vi "USB2XXX_LIN_Test.vi"() -> ()   [LabVIEW 2010]
panel:
  out "write return":i32
  out "pLINMsg out":T1
  out "read return":i32
  in  "pLINWiteMsg":T1={"ID"=2, "DataLen"=8, "Data[0]"=1, "Data[1]"=0, "Data[2]"=0, "Data[3]"=0, "Data[4]"=0, "Data[5]"=0, "Data[6]"=0, "Data[7]"=0, "Data[8]"=8}
  in  "pConfig":T2={"BaudRate"=19200, "CheckMode"=1, "MasterMode"=1, "BreakBits"=13}
  in  "Channel Index":u8(ring) items=["CH0"]
  in  "Device Index":i32(ring) items=["0", "1", "2", "3", "4", "5"]
  out "Flag(T:Write;F:Read)":bool=TRUE
  in  "stop":bool
  in  "Read":bool
  in  "Write":bool
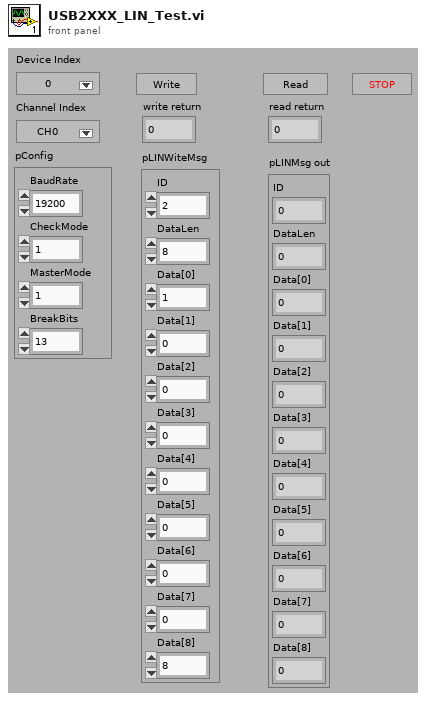
[diagram p1: front panel]
types:
  T1 = cluster{"ID":u8, "DataLen":u8, "Data[0]":u8, "Data[1]":u8, "Data[2]":u8, "Data[3]":u8, "Data[4]":u8, "Data[5]":u8, "Data[6]":u8, "Data[7]":u8, "Data[8]":u8}
  T2 = cluster{"BaudRate":u32, "CheckMode":u8, "MasterMode":u8, "BreakBits":u8}
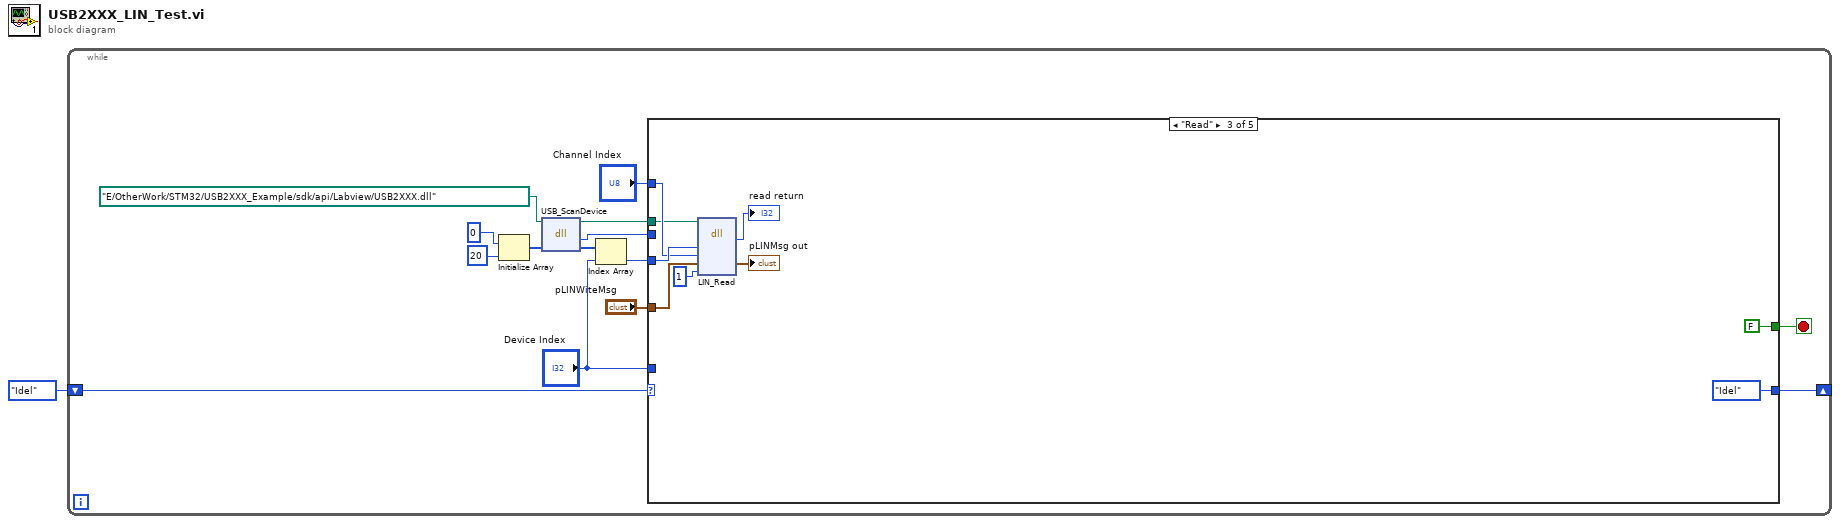
[diagram p0: block diagram]
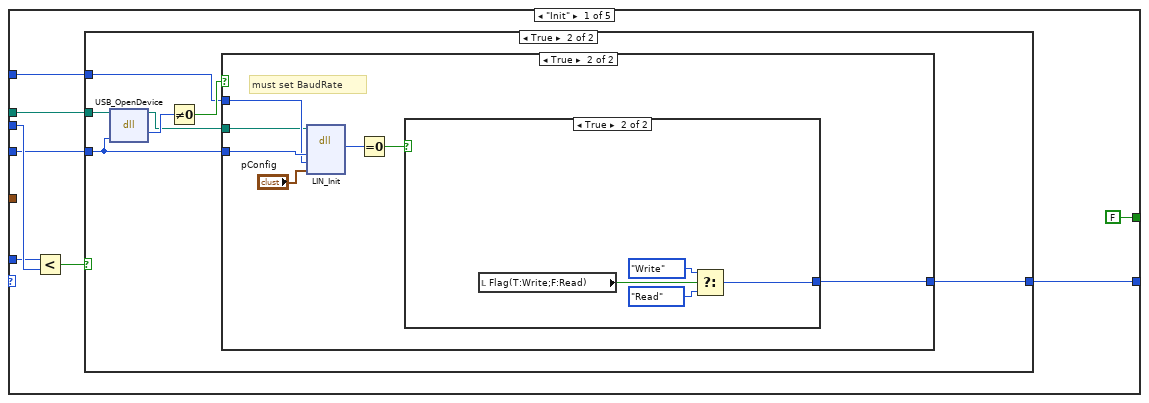
[diagram p2: hidden frame]
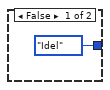
[diagram p3: hidden frame]
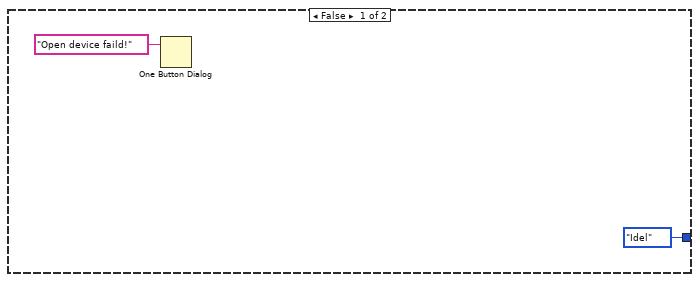
[diagram p4: hidden frame]
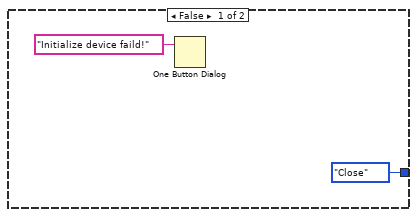
[diagram p5: hidden frame]
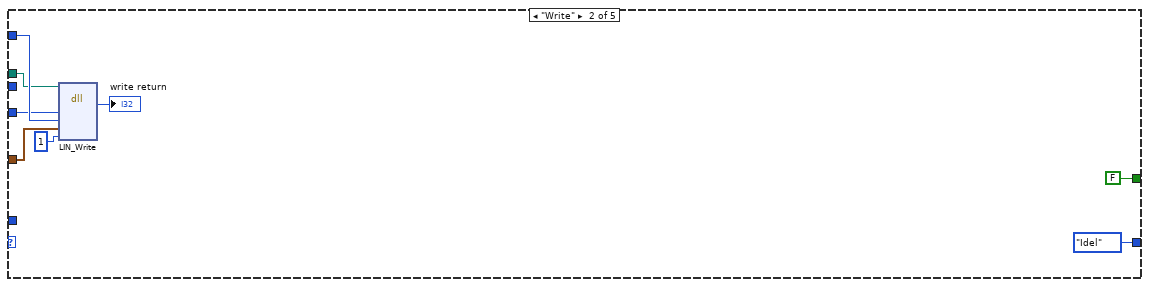
[diagram p6: hidden frame]
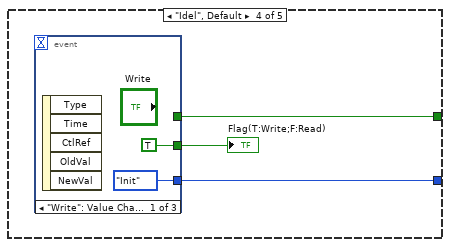
[diagram p7: hidden frame]
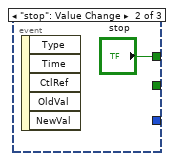
[diagram p8: hidden frame]
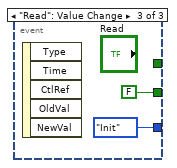
[diagram p9: hidden frame]
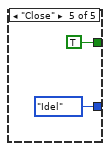
[diagram p10: hidden frame]
diagram:
  n1 = while {
    shift-right: [w14] -> _
    shift-left: enum16{"Init", "Write", "Read", "Idel", "Close"}."Idel" ("Enum") -> [w15]
    stop <- w12 stop-if-true
    n2 = Initialize Array(0, 20 ("dimension size")) -> (w11:i32[])
    n3 = dll-call lib="F:/OtherWork/STM32/USB2XXX_Example/trunk/Labview/PublicFiles/USB2XXX.*" fn="USB_ScanDevice"(path in=path "E:/OtherWork/STM32/USB2XXX_Example/sdk/api/Labview/USB2XXX.dll", "pDevNum"=w11) -> (path out=w2:path, "return type"=w6:i32, "pDevNum"=w8:i32[])  [unwired: 2 in, 1 out]
    n4 = Index Array(array=w8, index="Device Index") -> (element=w7:i32)
    n5 = case shown="\"Read\"" w15 {
      tunnel: [w22 enum16{"Init", "Write", "Read", "Idel", "Close"}."Idel" ("Enum") enum16{"Init", "Write", "Read", "Idel", "Close"}."Idel" ("Enum") w64 enum16{"Init", "Write", "Read", "Idel", "Close"}."Idel" ("Enum")] -> w14
      tunnel: w7 -> [w18 w50 w59 _ _]
      tunnel: "Channel Index" -> [w21 w51 w58 _ _]
      tunnel: [FALSE FALSE FALSE w65 TRUE] -> w12
      tunnel: w6 -> [w19 _ _ _ _]
      tunnel: "Device Index" -> [w17 _ _ _ _]
      tunnel: "pLINWiteMsg" -> [_ w49 w57 _ _]
      tunnel: w2 -> [w16 w47 w55 _ _]
      frame "Init" {
        n6 = Less?(x=w17, y=w19) -> (x < y?=w23:bool)
        n7 = case shown="True" w23 {
          tunnel: w18 -> [_ w28]
          tunnel: w21 -> [_ w29]
          tunnel: [enum16{"Init", "Write", "Read", "Idel", "Close"}."Idel" ("Enum") w27] -> w22
          tunnel: w16 -> [_ w26]
          frame False {
          }
          frame True {
            n8 = dll-call lib="F:/OtherWork/STM32/USB2XXX_Example/trunk/Labview/PublicFiles/USB2XXX.*" fn="USB_OpenDevice"(path in=w26, "DevIndex"=w28) -> (path out=w25:path, "return type"=w31:u8)  [unwired: 3 in, 1 out]
            n9 = Not Equal To 0?(x=w31) -> (x != 0?=w30:bool)
            n10 = case shown="True" w30 {
              tunnel: w29 -> [_ w37]
              tunnel: w28 -> [_ w38]
              tunnel: [enum16{"Init", "Write", "Read", "Idel", "Close"}."Idel" ("Enum") w39] -> w27
              tunnel: w25 -> [_ w35]
              frame False {
                n11 = One Button Dialog(message="Open device faild!") -> ()  [unwired: 1 in, 1 out]
              }
              frame True {
                # "must set BaudRate"
                n12 = dll-call lib="F:/OtherWork/STM32/USB2XXX_Example/trunk/Labview/PublicFiles/USB2XXX.*" fn="LIN_Init"(path in=w35, "DevHandle"=w38, "LINIndex"=w37, "pConfig"="pConfig") -> ("return type"=w36:i32)  [unwired: 5 in, 2 out]
                n13 = Equal To 0?(x=w36) -> (x = 0?=w40:bool)
                n14 = case shown="True" w40 {
                  tunnel: [enum16{"Init", "Write", "Read", "Idel", "Close"}."Close" ("Enum") w43] -> w39
                  frame False {
                    n15 = One Button Dialog(message="Initialize device faild!") -> ()  [unwired: 1 in, 1 out]
                  }
                  frame True {
                    n16 = local read "Flag(T:Write;F:Read)"() -> (w46:bool)
                    n17 = Select(t=enum16{"Init", "Write", "Read", "Idel", "Close"}."Write" ("Enum"), s=w46, f=enum16{"Init", "Write", "Read", "Idel", "Close"}."Read" ("Enum")) -> (s? t:f=w43:enum16{"Init", "Write", "Read", "Idel", "Close"})
                  }
                }
              }
            }
          }
        }
      }
      frame "Write" {
        n18 = dll-call lib="F:/OtherWork/STM32/USB2XXX_Example/trunk/Labview/PublicFiles/USB2XXX.*" fn="LIN_Write"(path in=w47, "DevHandle"=w50, "LINIndex"=w51, "pLINMsg"=w49, "Len"=u32 1) -> ("return type"=→"write return":i32)  [unwired: 6 in, 2 out]
      }
      frame "Read" {
        n19 = dll-call lib="F:/OtherWork/STM32/USB2XXX_Example/trunk/Labview/PublicFiles/USB2XXX.*" fn="LIN_Read"(path in=w55, "DevHandle"=w59, "LINIndex"=w58, "pLINMsg"=w57, "Len"=u32 1) -> ("return type"=→"read return":i32, "pLINMsg"=→"pLINMsg out":T1)  [unwired: 5 in, 2 out]
      }
      frame "Idel", Default {
        n20 = event shown="[0] \"Write\": Value Change" {
          selector: _ -> [_ _ _]
          dyn-events: _ -> [_ _ _]
          timeout: _ -> [_ _ _]
          tunnel: [TRUE _ FALSE] -> w66
          tunnel: [_ "stop" _] -> w65
          tunnel: [enum16{"Init", "Write", "Read", "Idel", "Close"}."Init" ("Enum") _ enum16{"Init", "Write", "Read", "Idel", "Close"}."Init" ("Enum")] -> w64
          event "Write": Value Change {
            n21 = event-data() -> ()  [unwired: 1 in, 5 out]
          }
          event "stop": Value Change {
            n22 = event-data() -> ()  [unwired: 1 in, 5 out]
          }
          event "Read": Value Change {
            n23 = event-data() -> ()  [unwired: 1 in, 5 out]
          }
        }
        "Flag(T:Write;F:Read)" <- w66
      }
      frame "Close" {
      }
    }
  }
